vi "l_matr_v3.vi"() -> ()   [LabVIEW 2009]
panel:
  in  "Index cifra":u8(knob)=4 scale=0.0..9.0
  in  "Tablou  3D":bool[][][](array[boolean])=[[[FALSE, TRUE, TRUE, TRUE, FALSE], [TRUE, FALSE, FALSE, FALSE, TRUE], [TRUE, FALSE, FALSE, FALSE, TRUE], [TRUE, FALSE, FALSE, FALSE, TRUE], [TRUE, FALSE, FALSE, FALSE, TRUE], [TRUE, FALSE, FALSE, FALSE, TRUE], [FALSE, TRUE, TRUE, TRUE, FALSE]], [[FALSE, FALSE, TRUE, FALSE, FALSE], [FALSE, TRUE, TRUE, FALSE, FALSE], [TRUE, FALSE, TRUE, FALSE, FALSE], [FALSE, FALSE, TRUE, FALSE, FALSE], [FALSE, FALSE, TRUE, FALSE, FALSE], [FALSE, FALSE, TRUE, FALSE, FALSE], [FALSE, FALSE, TRUE, FALSE, FALSE]], [[FALSE, TRUE, TRUE, TRUE, FALSE], [TRUE, FALSE, FALSE, FALSE, TRUE], [FALSE, FALSE, FALSE, FALSE, TRUE], [FALSE, FALSE, FALSE, TRUE, FALSE], [FALSE, FALSE, TRUE, FALSE, FALSE], [FALSE, TRUE, FALSE, FALSE, FALSE], [TRUE, TRUE, TRUE, TRUE, TRUE]], [[FALSE, TRUE, TRUE, TRUE, FALSE], [TRUE, FALSE, FALSE, FALSE, TRUE], [FALSE, FALSE, FALSE, FALSE, TRUE], [FALSE, FALSE, TRUE, TRUE, FALSE], [FALSE, FALSE, FALSE, FALSE, TRUE], [TRUE, FALSE, FALSE, FALSE, TRUE], [FALSE, TRUE, TRUE, TRUE, FALSE]], [[TRUE, FALSE, FALSE, FALSE, FALSE], [TRUE, FALSE, FALSE, FALSE, FALSE], [TRUE, FALSE, FALSE, TRUE, FALSE], [TRUE, TRUE, TRUE, TRUE, TRUE], [FALSE, FALSE, FALSE, TRUE, FALSE], [FALSE, FALSE, FALSE, TRUE, FALSE], [FALSE, FALSE, FALSE, TRUE, FALSE]], [[TRUE, TRUE, TRUE, TRUE, TRUE], [TRUE, FALSE, FALSE, FALSE, FALSE], [TRUE, TRUE, TRUE, TRUE, FALSE], [FALSE, FALSE, FALSE, FALSE, TRUE], [FALSE, FALSE, FALSE, FALSE, TRUE], [TRUE, FALSE, FALSE, FALSE, TRUE], [FALSE, TRUE, TRUE, TRUE, FALSE]], [[FALSE, TRUE, TRUE, TRUE, FALSE], [TRUE, FALSE, FALSE, FALSE, FALSE], [TRUE, FALSE, FALSE, FALSE, FALSE], [TRUE, TRUE, TRUE, TRUE, FALSE], [TRUE, FALSE, FALSE, FALSE, TRUE], [TRUE, FALSE, FALSE, FALSE, TRUE], [FALSE, TRUE, TRUE, TRUE, FALSE]], [[TRUE, TRUE, TRUE, TRUE, TRUE], [FALSE, FALSE, FALSE, FALSE, TRUE], [FALSE, FALSE, FALSE, FALSE, TRUE], [FALSE, FALSE, FALSE, TRUE, FALSE], [FALSE, FALSE, TRUE, FALSE, FALSE], [FALSE, TRUE, FALSE, FALSE, FALSE], [TRUE, FALSE, FALSE, FALSE, FALSE]], [[FALSE, TRUE, TRUE, TRUE, FALSE], [TRUE, FALSE, FALSE, FALSE, TRUE], [TRUE, FALSE, FALSE, FALSE, TRUE], [FALSE, TRUE, TRUE, TRUE, FALSE], [TRUE, FALSE, FALSE, FALSE, TRUE], [TRUE, FALSE, FALSE, FALSE, TRUE], [FALSE, TRUE, TRUE, TRUE, FALSE]], [[FALSE, TRUE, TRUE, TRUE, FALSE], [TRUE, FALSE, FALSE, FALSE, TRUE], [TRUE, FALSE, FALSE, FALSE, TRUE], [FALSE, TRUE, TRUE, TRUE, TRUE], [FALSE, FALSE, FALSE, FALSE, TRUE], [FALSE, FALSE, FALSE, FALSE, TRUE], [FALSE, TRUE, TRUE, TRUE, FALSE]]]
  out "Linia selectata":bool[](array[boolean])=[TRUE, FALSE, FALSE, FALSE, FALSE]
  out "Array 3":bool[][](array[boolean])=[[TRUE, FALSE, FALSE, FALSE, FALSE], [TRUE, FALSE, FALSE, FALSE, FALSE], [TRUE, FALSE, FALSE, TRUE, FALSE], [TRUE, TRUE, TRUE, TRUE, TRUE], [FALSE, FALSE, FALSE, TRUE, FALSE], [FALSE, FALSE, FALSE, TRUE, FALSE], [FALSE, FALSE, FALSE, TRUE, FALSE]]
  out "Linia":u8(slide)=1 scale=6.0..0.0
  in  "Iesire":bool
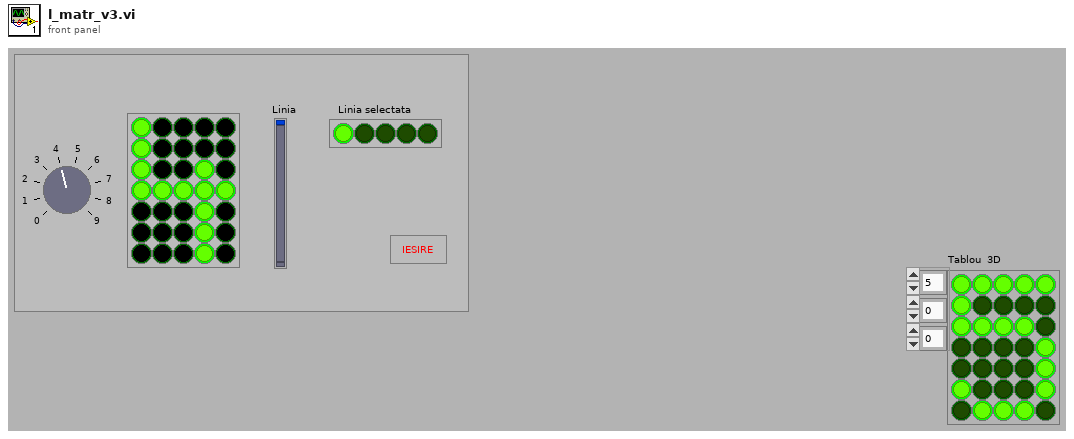
[diagram p1: front panel]
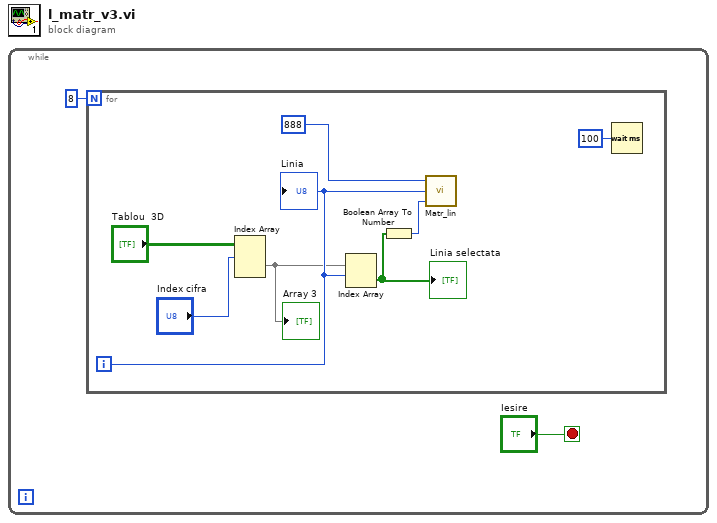
[diagram p0: block diagram]
diagram:
  n1 = while {
    stop <- "Iesire" stop-if-true
    n2 = for {
      N: 8 -> [_]
      i -> [w6]
      n3 = Index Array(array="Tablou  3D", index (dim 0)="Index cifra") -> (element=w3:bool[][])  [unwired: 2 in]
      "Array 3" <- w3
      n4 = Index Array(array=w3, index (row)=w6) -> (element=w7:bool[])  [unwired: 1 in]
      "Linia selectata" <- w7
      n5 = Boolean Array To Number(Boolean array=w7) -> (number=w8:u32)
      n6 = call "Matr_lin.vi"("Date"=w8, "Linia"=w6, "Adresa port paralel"=888) -> ()  [unwired: 2 out]
      n7 = Wait (ms)(milliseconds to wait=u32 100) -> ()  [unwired: 1 out]
      "Linia" <- w6
    }
  }
